vi "Teleop Drivetrain Control.vi"(10 "Driver Axes":T1, 11 "Driver Buttons":T2) -> ()   [LabVIEW 2013]
uses:
  <vilib>/Rock Robotics/WPI/Joystick/WPI_JoystickButtonState.ctl
  Drivetrain Control.ctl
  DT Mode.ctl
  Common Code/Change Detect Boolean.vi
  <vilib>/Analysis/coordinate.llb/2D Cartesian Coordinate Rotation (Scalar).vi
  Utilities/Vector Magnitude.vi
  Robot Global Data.vi
  <vilib>/Rock Robotics/WPI/Gyro/WPI_GyroRefNum Registry Get.vi
  <vilib>/Rock Robotics/WPI/Gyro/WPI_GyroGetAngle.vi
  <vilib>/Analysis/NI_AALPro.lvlib
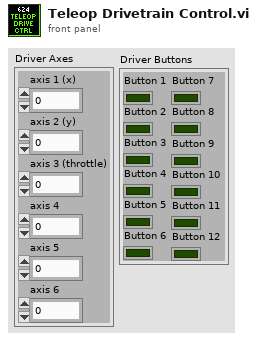
[diagram p1: front panel]
types:
  T1 = cluster{"axis 1 (x)":dbl, "axis 2 (y)":dbl, "axis 3 (throttle)":dbl, "axis 4":dbl, "axis 5":dbl, "axis 6":dbl}
  T2 = typedef "WPI_JoystickButtonState.ctl" = cluster{"Button 1":bool, "Button 2":bool, "Button 3":bool, "Button 4":bool, "Button 5":bool, "Button 6":bool, "Button 7":bool, "Button 8":bool, "Button 9":bool, "Button 10":bool, "Button 11":bool, "Button 12":bool}
  T3 = typedef "Drivetrain Control.ctl" = cluster{"axis 1 (x)":dbl, "axis 2 (y)":dbl, "Mode":T4, "heading target":dbl, "steer axis":dbl, "omni?":bool, "Low Gear?":bool, "distance target":cluster{"x":dbl, "y":dbl}, "PID Params":cluster{"X Dist":cluster{"PID gains":cluster{"proportional gain (Kc)":dbl, "integral time (Ti, min)":dbl, "derivative time (Td, min)":dbl}, "output range":cluster{"output high":dbl, "output low":dbl}}, "Y Dist":cluster{"PID gains":cluster{"proportional gain (Kc)":dbl, "integral time (Ti, min)":dbl, "derivative time (Td, min)":dbl}, "output range":cluster{"output high":dbl, "output low":dbl}}}, "Coast":bool}
  T4 = typedef "DT Mode.ctl" = enum16{"Manual", "Gyro Steer", "Distance Drive", "Fieldcentric", "Roll Maneuver", "Alt Roll Maneuver"}
  T5 = typedef "Dashboard UDP Packet.ctl" = cluster{"Camera":T6, "Gyro":T7, "Encoder":T9, "Auto Shift":T10, "Auton":T11, "Drive/Ramp X":dbl, "Drive/Ramp Y":dbl, "Drive/Battery Cutoff":dbl, "Pressure/Compressor Min Voltage":dbl, "Pressure/Compressor Delay":dbl, "Controller/Strafe Correction":bool, "Shooter":T12, "Rollers":T13, "Abort":bool, "Finish":bool, "IR Halo Sustain Time":dbl, "Disable Compressor":bool, "Center Omni Drive Delay":i32, "Vision Mode":T14, "Radius Throttle":bool, "Fieldcentric":T15, "Roll":T16, "Stick Deadband":dbl}
  T6 = typedef "Camera Controls.ctl" = cluster{"Camera/View Angle X":dbl, "Camera/Goal Track Timeout":dbl, "Camera/View Angle Y":dbl, "Camera/Goal Exposure":dbl, "Camera/Vision Receive Timeout":dbl, "Camera/Offset 1":dbl, "Camera/Offset 2":dbl}
  T7 = typedef "Gyro Controls.ctl" = cluster{"Gyro/Angle Tolerance":dbl, "Gyro/Steer Closeness Threshold":dbl, "Steer PID":T8, "Steer Close PID":T8}
  T8 = typedef "PID Params.ctl" = cluster{"max":dbl, "min":dbl, "P":dbl, "I":dbl, "D":dbl}
  T9 = typedef "Encoder Controls.ctl" = cluster{"Encoders/Reset":bool, "Encoders/Omni Constant":dbl, "Encoders/Omni Tick Constant":dbl, "Encoders/Left Constant":dbl, "Encoders/Right Constant":dbl, "Encoders/Right Tick Constant":dbl}
  T10 = typedef "Auto Shift Controls.ctl" = cluster{"AutoShift/Upshift Throttle Accel":dbl, "AutoShift/Speed Threshold":dbl, "AutoShift/Upshift Throttle":dbl, "AutoShift/Upshift Accel":dbl, "AutoShift/Downshift Accel":dbl, "AutoShift/Downshift Throttle":dbl, "AutoShift/Delay":dbl, "AutoShift/Enabled":bool}
  T11 = typedef "Auton Controls.ctl" = cluster{"Auton/Left Shoot X-Coord":dbl, "Auton/Right Shoot X-Coord":dbl, "DistDrive/Distance Stop Threshold":dbl, "DistDrive/Max Stop Speed":dbl, "Auton/Back Piston Time":dbl, "Auton/Manual Hot":bool, "Auton/Manual Hot Right":bool, "Default X PID":T8, "Default Y PID":T8}
  T12 = typedef "Shooter Controls.ctl" = cluster{"Shooter/Reset Time":dbl, "Shooter/Release Delay":dbl, "Shooter/Pressure Steady Time":dbl, "Shooter/Misfire Delay":dbl, "Shooter/Ball Settle Time":dbl, "Shooter/Line IR Delay":dbl, "Pressure/Upper PSI Time":dbl, "Pressure/Lower PSI Time":dbl, "Shooter/Punch Delay":dbl, "Shooter/Target Pressure":dbl, "Pressure/Line B":dbl, "Pressure/Line M":dbl, "Pressure/Shooter M":dbl, "Pressure/Shooter B":dbl, "Halo Time":dbl, "Soft Release Delay":dbl, "Soft Unpin Delay":dbl, "Soft Shoot Delay":dbl}
  T13 = typedef "Roller Controls.ctl" = cluster{"Roller/Load IRs Verify Time":dbl, "Roller/Center IR Latch Time":dbl, "Roller/Speed Front":dbl, "Roller/Speed Back":dbl, "Roller/Entry Timeout":dbl, "Roller/To Center Timeout":dbl, "Roller/Sustain Time":dbl, "Roller/Verify Center Time":dbl}
  T14 = typedef "Vision Mode.ctl" = enum16{"Normal", "Extreme Left", "Extreme Right"}
  T15 = typedef "Fieldcentric Controls.ctl" = cluster{"Relative Angle":bool, "Point Robot":bool, "X/Y ratio low":dbl, "Steering Gain":dbl, "Force Omni Down":bool, "Enable":bool, "X/Y ratio high":dbl}
  T16 = typedef "Roll Maneuver.ctl" = cluster{"X 1":dbl, "Y 1":dbl, "Y 2":dbl, "X 2":dbl, "Y 3":dbl, "X 3":dbl, "Time 1":i32, "Time 2":i32, "Time 3":i32, "Angle Start":dbl, "Angle End":dbl, "Angle Linearity":dbl}
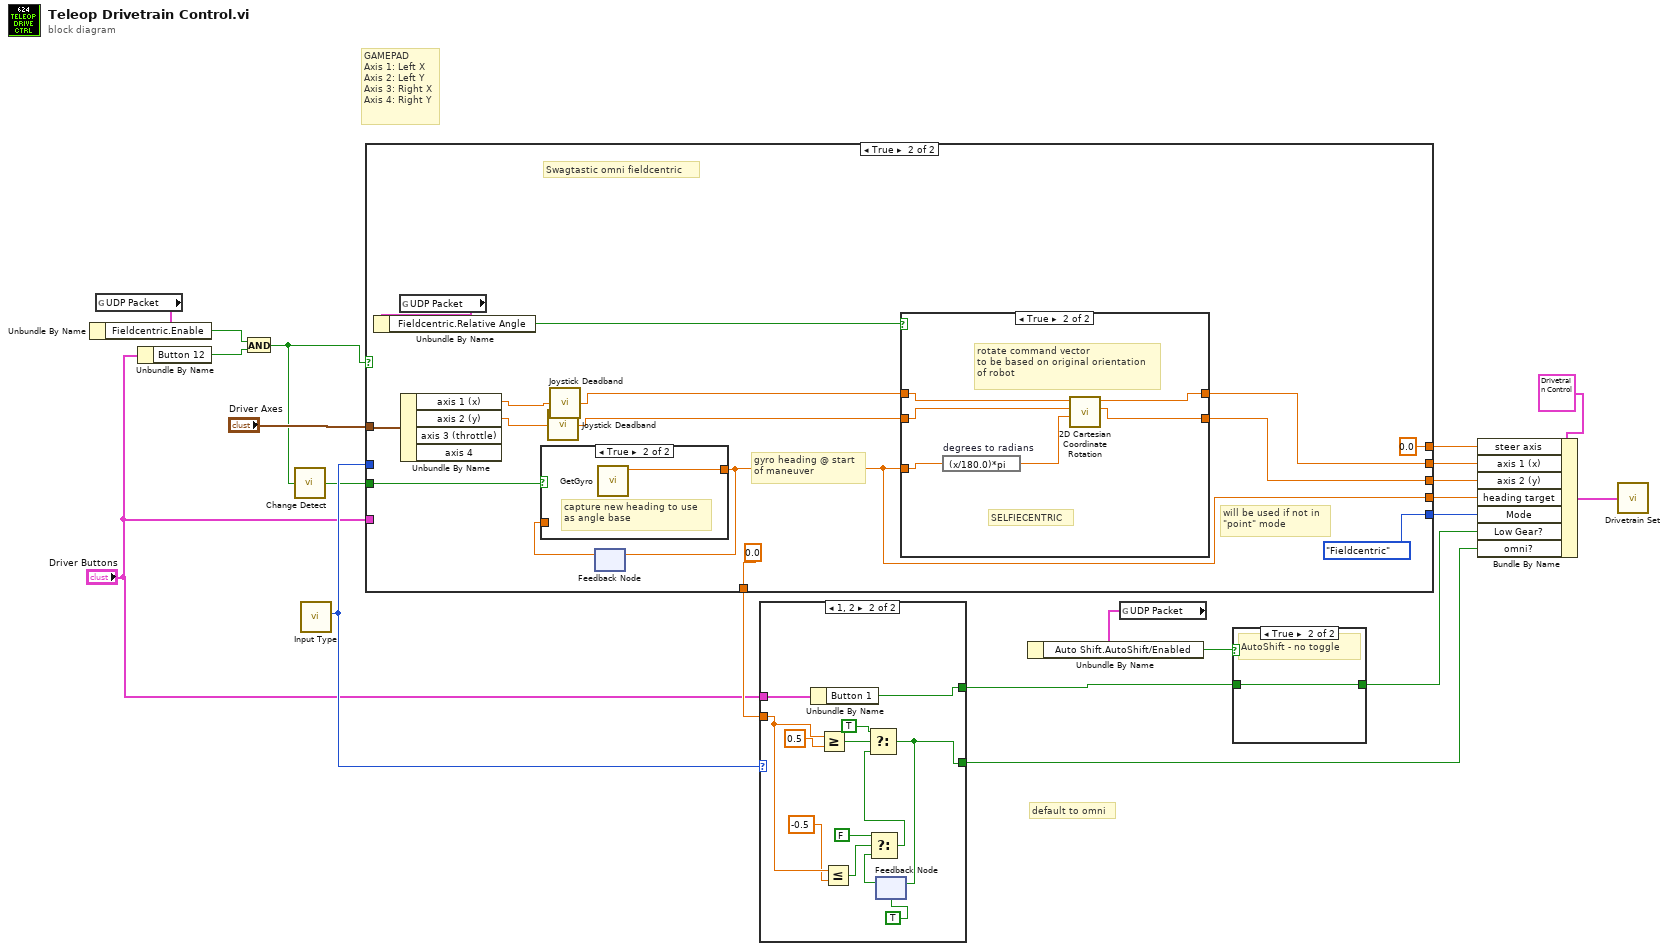
[diagram p0: block diagram]
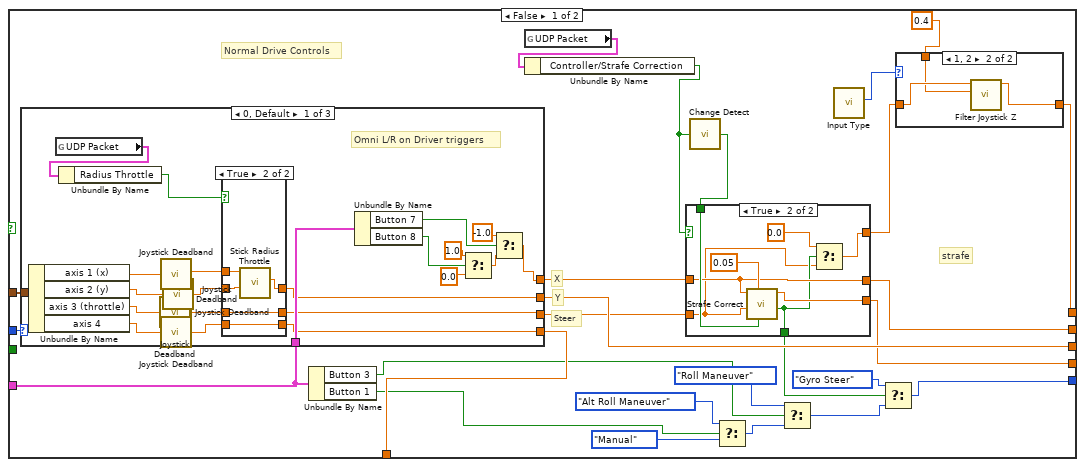
[diagram p2: hidden frame]
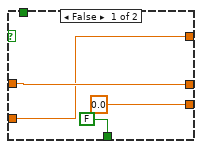
[diagram p3: hidden frame]
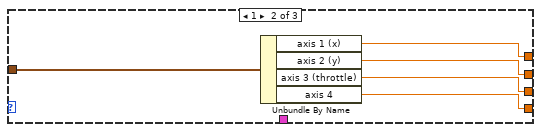
[diagram p5: hidden frame]
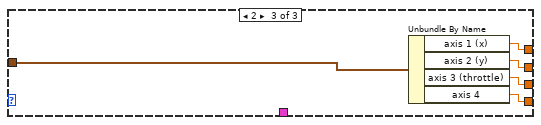
[diagram p6: hidden frame]
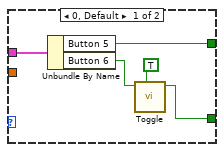
[diagram p10: hidden frame]
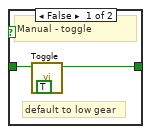
[diagram p11: hidden frame]
diagram:
  # "GAMEPAD\nAxis 1: Left X\nAxis 2: Left Y\nAxis 3: Right X\nAxis 4: Right Y"
  # "default to omni"
  n1 = global read "Robot Global Data.vi" "UDP Packet"() -> (w5:T5)
  n2 = Unbundle By Name(w5) -> ("Fieldcentric.Enable"=w4:bool)
  n3 = Unbundle By Name("Driver Buttons") -> ("Button 12"=w3:bool)
  n4 = And(x=w4, y=w3) -> (x .and. y?=w2:bool)
  n5 = call-poly "Change Detect.vi"("In"=w2) -> ("Changed?"=w1:bool)
  n6 = call "Input Type.vi"() -> ("Mode"=w15:i32)  [unwired: 11 in]
  n7 = case shown="True" w2 {
    tunnel: "Driver Axes" -> [w47 w116]
    tunnel: [w46 0.0 ("axis 4")] -> w20
    tunnel: [w45 w113] -> w19
    tunnel: [w44 0.0 ("Z Out")] -> w18
    tunnel: w15 -> [w43 _]
    tunnel: [w35 w109] -> w9
    tunnel: [w34 w114] -> w8
    tunnel: [w30 DT_Mode."Fieldcentric" ("t")] -> w7
    tunnel: "Driver Buttons" -> [w29 _]
    tunnel: w1 -> [_ w110]
    frame False {
      # "Normal Drive Controls"
      # "Steer"
      # "Y"
      # "X"
      # "strafe"
      n8 = case shown="0, Default" w43 {
        tunnel: [w63 w91 w96] -> w41
        tunnel: [w80 w93 w98] -> w38
        tunnel: [w70 w92 w97] -> w45
        tunnel: [w60 w90 w95] -> w46
        tunnel: w47 -> [w81 w94 w99]
        tunnel: w29 -> [w79 _ _]
        frame 0, Default {
          # "Omni L/R on Driver triggers"
          n9 = Unbundle By Name(w81) -> ("axis 1 (x)"=w69:dbl, "axis 2 (y)"=w67:dbl, "axis 3 (throttle)"=w65:dbl, "axis 4"=w62:dbl)
          n10 = global read "Robot Global Data.vi" "UDP Packet"() -> (w72:T5)
          n11 = Unbundle By Name(w72) -> ("Radius Throttle"=w71:bool)
          n12 = call "Joystick Deadband.vi"() -> ()  [unwired: 1 in, 1 out]
          n13 = call "Joystick Deadband.vi"("Stick In"=w69) -> ("Stick Out"=w68:dbl)
          n14 = call "Joystick Deadband.vi"("Stick In"=w65) -> ("Stick Out"=w64:dbl)
          n15 = call "Joystick Deadband.vi"("Stick In"=w62) -> ("Stick Out"=w61:dbl)
          n16 = call "Joystick Deadband.vi"("Stick In"=w67) -> ("Stick Out"=w66:dbl)
          n17 = case shown="True" w71 {
            tunnel: w66 -> [w84 w88]
            tunnel: [w84 w87] -> w70
            tunnel: w68 -> [_ w89]
            tunnel: w64 -> [w83 w86]
            tunnel: [w83 w86] -> w63
            tunnel: w61 -> [w82 w85]
            tunnel: [w82 w85] -> w60
            frame False {
            }
            frame True {
              n18 = call "Stick Radius Throttle.vi"("Stick Y"=w88, "Stick X"=w89) -> ("Throttle"=w87:dbl)  [unwired: 9 in]
            }
          }
          n19 = Unbundle By Name(w79) -> ("Button 7"=w76:bool, "Button 8"=w77:bool)
          n20 = Select(t=1.0, s=w77, f=0.0 ("t")) -> (s? t:f=w78:dbl)
          n21 = Select(t=-1.0, s=w76, f=w78) -> (s? t:f=w80:dbl)
        }
        frame 1 {
          n22 = Unbundle By Name(w94) -> ("axis 1 (x)"=w93:dbl, "axis 2 (y)"=w92:dbl, "axis 3 (throttle)"=w91:dbl, "axis 4"=w90:dbl)
        }
        frame 2 {
          n23 = Unbundle By Name(w99) -> ("axis 1 (x)"=w98:dbl, "axis 2 (y)"=w97:dbl, "axis 3 (throttle)"=w96:dbl, "axis 4"=w95:dbl)
        }
      }
      n24 = Unbundle By Name(w29) -> ("Button 3"=w22:bool, "Button 1"=w23:bool)
      n25 = global read "Robot Global Data.vi" "UDP Packet"() -> (w40:T5)
      n26 = Unbundle By Name(w40) -> ("Controller/Strafe Correction"=w37:bool)
      n27 = call-poly "Change Detect.vi"("In"=w37) -> ("Changed?"=w36:bool)
      n28 = case shown="True" w37 {
        tunnel: [w51 w57] -> w34
        tunnel: w41 -> [w48 w53]
        tunnel: w38 -> [w51 w57]
        tunnel: w36 -> [_ w58]
        tunnel: [0.0 ("Angle Target") w56] -> w35
        tunnel: [FALSE ("Correction Active") w55] -> w32
        tunnel: [w48 w52] -> w33
        frame False {
        }
        frame True {
          n29 = call "Strafe Correct.vi"("Reset"=w58, "Max Steer"=0.05, "Steer In"=w53, "X In"=w57) -> ("Correction Active"=w55:bool, "Angle Target"=w56:dbl)  [unwired: 6 in]
          n30 = Select(t=0.0 ("axis 3 (throttle)"), s=w55, f=w53) -> (s? t:f=w52:dbl)
        }
      }
      n31 = Select(t=DT_Mode."Alt Roll Maneuver", s=w23, f=DT_Mode."Manual" ("t")) -> (s? t:f=w24:T4)
      n32 = Select(t=DT_Mode."Roll Maneuver", s=w22, f=w24) -> (s? t:f=w27:T4)
      n33 = call "Input Type.vi"() -> ("Mode"=w42:i32)  [unwired: 11 in]
      n34 = Select(t=DT_Mode."Gyro Steer", s=w32, f=w27) -> (s? t:f=w30:T4)
      n35 = case shown="1, 2" w42 {
        tunnel: w33 -> [w100 w102]
        tunnel: [w100 w103] -> w44
        tunnel: 0.4 -> [_ w101]
        frame 0, Default {
        }
        frame 1, 2 {
          n36 = call "Filter Joystick Z.vi"("Scale"=w101, "Z In"=w102) -> ("Z Out"=w103:dbl)  [unwired: 9 in]
        }
      }
    }
    frame True {
      # "will be used if not in\n\"point\" mode"
      # "gyro heading @ start\nof maneuver"
      # "Swagtastic omni fieldcentric"
      n37 = global read "Robot Global Data.vi" "UDP Packet"() -> (w117:T5)
      n38 = Unbundle By Name(w117) -> ("Fieldcentric.Relative Angle"=w115:bool)
      n39 = Unbundle By Name(w116) -> ("axis 1 (x)"=w107:dbl, "axis 2 (y)"=w105:dbl)  [unwired: 2 out]
      n40 = call "Joystick Deadband.vi"("Stick In"=w105) -> ("Stick Out"=w104:dbl)
      n41 = call "Joystick Deadband.vi"("Stick In"=w107) -> ("Stick Out"=w106:dbl)
      n42 = feedback #1() -> (w111:dbl)  [unwired: 1 in]
      n43 = case shown="True" w110 {
        tunnel: [w119 w120] -> w109
        tunnel: w111 -> [w119 _]
        frame False {
          # "middle of maneuver, keep old \ngyro frame of reference"
        }
        frame True {
          # "capture new heading to use\nas angle base"
          n44 = call "GetGyro.vi"() -> ("Angle"=w120:dbl)  [unwired: 9 in, 2 out]
        }
      }
      n45 = feedback-in #1(w109) -> ()
      n46 = case shown="True" w115 {
        tunnel: w106 -> [w122 w128]
        tunnel: w104 -> [w121 w127]
        tunnel: [w122 w126] -> w114
        tunnel: [w121 w125] -> w113
        tunnel: w109 -> [_ w124]
        frame False {
          # "just use field frame of reference\nno fancy maneuver stuff"
        }
        frame True {
          # "SELFIECENTRIC"
          # "rotate command vector\nto be based on original orientation\nof robot"
          n47 = expression code="(x/180.0)*pi" "degrees to radians"(w124) -> (w123:dbl)
          n48 = call-poly <vilib>:"2D Cartesian Coordinate Rotation.vi"("theta"=w123, "y"=w127, "x"=w128) -> ("y out"=w125:dbl, "x out"=w126:dbl)  [unwired: 6 in, 1 out]
        }
      }
    }
  }
  n49 = case shown="1, 2" w15 {
    tunnel: [w133 w135] -> w13
    tunnel: "Driver Buttons" -> [w132 w145]
    tunnel: [w131 w144] -> w17
    tunnel: w20 -> [_ w146]
    frame 0, Default {
      n50 = Unbundle By Name(w132) -> ("Button 5"=w133:bool, "Button 6"=w130:bool)
      n51 = call "Toggle.vi"("Initial Value"=TRUE, "In"=w130) -> ("Toggled"=w131:bool)  [unwired: 9 in]
    }
    frame 1, 2 {
      n52 = Unbundle By Name(w145) -> ("Button 1"=w135:bool)
      n53 = Greater Or Equal?(x=w146, y=0.5) -> (x >= y?=w140:bool)
      n54 = Less Or Equal?(x=w146, y=-0.5) -> (x <= y?=w141:bool)
      n55 = feedback #2(TRUE ("t")) -> (w142:bool)
      n56 = Select(t=FALSE, s=w141, f=w142) -> (s? t:f=w143:bool)
      n57 = Select(t=TRUE, s=w140, f=w143) -> (s? t:f=w144:bool)
      n58 = feedback-in #2(w144) -> ()
    }
  }
  n59 = global read "Robot Global Data.vi" "UDP Packet"() -> (w11:T5)
  n60 = Unbundle By Name(w11) -> ("Auto Shift.AutoShift/Enabled"=w10:bool)
  n61 = case shown="True" w10 {
    tunnel: [w149 w150] -> w14
    tunnel: w13 -> [w148 w150]
    frame False {
      # "default to low gear"
      # "Manual - toggle"
      n62 = call "Toggle.vi"("Initial Value"=TRUE, "In"=w148) -> ("Toggled"=w149:bool)  [unwired: 9 in]
    }
    frame True {
      # "AutoShift - no toggle"
    }
  }
  n63 = Bundle By Name(cluster=T3 {"axis 1 (x)"=0.0, "axis 2 (y)"=0.0, "Mode"=enum."Manual", "heading target"=0.0, "steer axis"=0.0, "omni?"=FALSE, "Low Gear?"=FALSE, "distance target"={"x"=0.0, "y"=0.0}, "PID Params"={"X Dist"={"PID gains"={"proportional gain (Kc)"=0.0, "integral time (Ti, min)"=0.0, "derivative time (Td, min)"=0.0}, "output range"={"output high"=0.0, "output low"=0.0}}, "Y Dist"={"PID gains"={"proportional gain (Kc)"=0.0, "integral time (Ti, min)"=0.0, "derivative time (Td, min)"=0.0}, "output range"={"output high"=0.0, "output low"=0.0}}}, "Coast"=FALSE} ("Drivetrain Control"), "steer axis"=w18, "axis 1 (x)"=w8, "axis 2 (y)"=w19, "heading target"=w9, "Mode"=w7, "Low Gear?"=w14, "omni?"=w17) -> (w16:T3)
  n64 = call "Drivetrain Set.vi"("Drivetrain Control"=w16) -> ()  [unwired: 1 in]
